vi "libssh2_sftp_rewind.vi"(8 "error in (no error)":errorcluster, 11 "sftp handle":T1) -> (0 "error out":errorcluster)   [LabVIEW 2013, in "libssh2.lvlib"]
doc: "Set the file position of a file handle to zero."
uses:
  libssh2.lvlib
  SFTP Handle Refnum.ctl
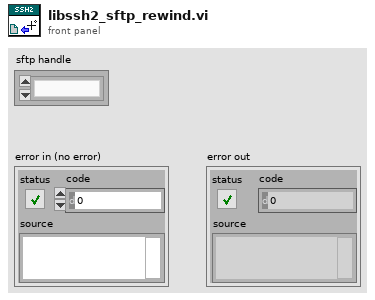
[diagram p1: front panel]
types:
  T1 = typedef "libssh2.lvlib/SFTP Handle Refnum.ctl" = refnum<k1>
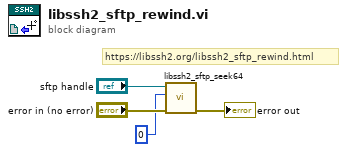
[diagram p0: block diagram]
diagram:
  # "https://libssh2.org/libssh2_sftp_rewind.html"
  n1 = call "libssh2_sftp_seek64.vi"("error in (no error)"="error in (no error)", "offset"=u64 0, "sftp handle"="sftp handle") -> ("error out"=→"error out":errorcluster)  [unwired: 8 in]
